vi "SECoP-updateParameter_2.vi"(6 "Timestamp":dbl=nan, 7 "sigma":string, 8 "error in (no error)":errorcluster, 9 "value":string, 10 "parameter name":string, 11 "DLL path (in)":T1) -> (0 "error out":errorcluster, 3 "DLL path (out)":T1)   [LabVIEW 2023, in "SECoP.lvlib"]
doc: "Call <b>\"SECoP-updateParameter_2.vi\"</b>, if you have a new value for an existing parameter (read- or writable). All clients which subscribed to this module should be informed about the new value.\n\n<b>DLL path</b> input and output of cluster from \"SECoP-Initialize.vi\"\n<b>parameter name</b> full name of parameter including node id and module name (format <b>node-id:module:parameter</b>)\n<b>value</b> new value of parameter as JSON string\n<b>sigma</b> if applicable, the error bar of the new value of parameter as JSON string\n<b>timestamp</b> time in seconds (with fraction) from 1970/1/1 0:0am of data (or NaN for actual time)"
uses:
  SECoP.lvlib
  SECoP-libraries.ctl
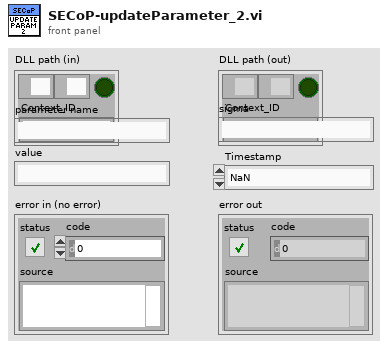
[diagram p1: front panel]
types:
  T1 = typedef "SECoP.lvlib/SECoP-libraries.ctl" = cluster{"serverDLL":path, "variantDLL":path, "cleanup_mode":bool, "Context_ID":string}
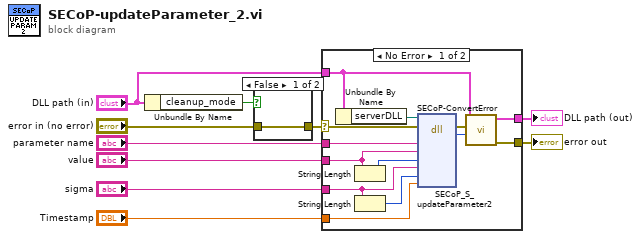
[diagram p0: block diagram]
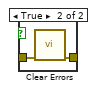
[diagram p2: hidden frame]
diagram:
  n1 = Unbundle By Name("DLL path (in)") -> ("cleanup_mode"=w7:bool)
  n2 = case shown="False" w7 {
    tunnel: "error in (no error)" -> [w11 w13]
    tunnel: [w11 w12] -> w5
    frame False {
    }
    frame True {
      n3 = call <vilib>:"Clear Errors.vi"("error in (no error)"=w13) -> ("error out"=w12:errorcluster)  [unwired: 5 in, 1 out]
    }
  }
  n4 = case shown="No Error" w5 {
    selector: w5 -> [w22 w27]
    tunnel: "DLL path (in)" -> [w15 w28]
    tunnel: [w25 w28] -> w10
    tunnel: [w26 w27] -> w9
    tunnel: "parameter name" -> [w21 _]
    tunnel: "Timestamp" -> [w20 _]
    tunnel: "value" -> [w18 _]
    tunnel: "sigma" -> [w17 _]
    frame No Error {
      n5 = Unbundle By Name(w15) -> ("serverDLL"=w14:path)
      n6 = String Length(string=w18) -> (length=w19:i32)
      n7 = String Length(string=w17) -> (length=w16:i32)
      n8 = dll-call lib="Z:/Praktische Aufgaben/SECoP-LabVIEW2015/32bit/SECoP32.dll" fn="SECoP_S_updateParameter2"(path in=w14, error in=w22, "ParameterName"=w21, "Value"=w18, "ValueSize"=w19, "Sigma"=w17, "SigmaSize"=w16, "Timestamp"=w20) -> (error out=w24:errorcluster, "return type"=w23:i32)  [unwired: 7 in, 1 out]
      n9 = call "SECoP-ConvertError.vi"("return code"=w23, "error in (no error)"=w24, "DLL path (in)"=w15) -> ("error out"=w26:errorcluster, "DLL path (out)"=w25:T1)  [unwired: 7 in]
    }
    frame Error {
    }
  }
  "DLL path (out)" <- w10
  "error out" <- w9
